vi "Arrange Controls in 2D Array.vi"(8 "error in (no error)":errorcluster, 11 "Controls[]":refnum<vi>[](array[refnum])) -> (0 "error out":errorcluster, 2 "controls 2D[]":refnum<vi>[][](array[refnum]), 3 "Controls[]":refnum<vi>[](array[refnum]))   [LabVIEW 2018, in "NISAST VI Scripting.lvlib" / "VI.lvlib" / "Front Panel.lvlib"]
uses:
  Front Panel.lvlib
  Connector/Connector.lvlib
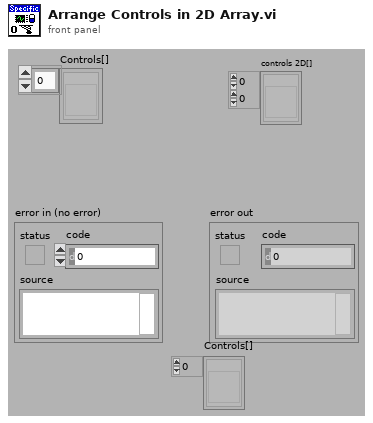
[diagram p1: front panel]
types:
  T1 = typedef "NISAST VI Scripting.lvlib/VI.lvlib/Front Panel.lvlib/Connector Pane Type.ctl" = enum16{"4-2-2-4", "5-2-2-2-5", "Others"}
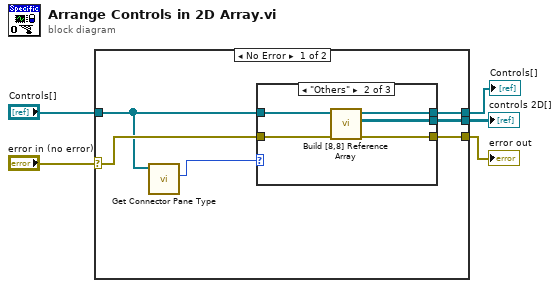
[diagram p0: block diagram]
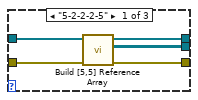
[diagram p2: hidden frame]
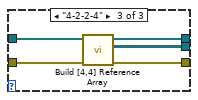
[diagram p3: hidden frame]
diagram:
  n1 = case shown="No Error" "error in (no error)" {
    selector: "error in (no error)" -> [w9 w28]
    tunnel: [w11 _] -> w3
    tunnel: [w10 w28] -> w5
    tunnel: "Controls[]" -> [w7 w27]
    tunnel: [w8 w27] -> w1
    frame No Error {
      n2 = call "Get Connector Pane Type.vi"("Controls[]"=w7) -> ("Connector Pane Type"=w6:T1)  [unwired: 1 in, 8 out]
      n3 = case shown="\"Others\"" w6 {
        tunnel: w7 -> [w13 w21 w23]
        tunnel: [w16 w18 w26] -> w11
        tunnel: w9 -> [w15 w20 w25]
        tunnel: [w14 w17 w24] -> w10
        tunnel: [w12 w19 w22] -> w8
        frame "5-2-2-2-5" {
          n4 = call "Build [5,5] Reference Array.vi"("error in"=w15, "controls references"=w13) -> ("error out"=w14:errorcluster, "2-D controls references array"=w16:refnum<vi>[][], "controls references out"=w12:refnum<vi>[])  [unwired: 1 in, 6 out]
        }
        frame "Others" {
          n5 = call "Build [8,8] Reference Array.vi"("error in"=w20, "controls references"=w21) -> ("error out"=w17:errorcluster, "2-D controls references array"=w18:refnum<vi>[][], "controls references out"=w19:refnum<vi>[])  [unwired: 7 out]
        }
        frame "4-2-2-4" {
          n6 = call "Build [4,4] Reference Array.vi"("error in"=w25, "controls references"=w23) -> ("error out"=w24:errorcluster, "2-D controls references array"=w26:refnum<vi>[][], "controls references out"=w22:refnum<vi>[])  [unwired: 1 in, 6 out]
        }
      }
    }
    frame Error {
    }
  }
  "error out" <- w5
  "controls 2D[]" <- w3
  "Controls[]" <- w1
